vi "testDMA_7858(chunk).vi"() -> ()   [LabVIEW 2020]
uses:
  <vilib>/rvi/Emulation/niFpgaGetClockAttributes.vi
  <vilib>/rvi/Emulation/niFpgaSctlEmulationGetInTimedLoop.vi
  <vilib>/rvi/Emulation/niFpgaEmulationReportErrorSimple.vi
  <vilib>/rvi/DataTransferAndStorage/Container/Common/niFpgaContainerExecOnDevCompGetState.vi
  <vilib>/rvi/errors/niFpgaSetErrorForExecOnDevCompSimple.vi
  <vilib>/rvi/eio/common/nirviEmuReportErrorAndStop.vi
  <vilib>/rvi/interface/RandomDataEmulation/nirviRandomDataAcquireLock.vi
  <vilib>/rvi/interface/RandomDataEmulation/nirviRandomDataQueueStore.vi
  <vilib>/rvi/interface/RandomDataEmulation/nirviRandomDataReleaseLock.vi
  <vilib>/rvi/interface/RandomDataEmulation/nirviFPGAContextMergeError.vi
  <vilib>/rvi/interface/RandomDataEmulation/nirviRandomDataCheckExitLoopConditions.vi
  <vilib>/express/rvi/timingcommon/nirviCommon.vi
  <vilib>/rvi/interface/RandomDataEmulation/niFpgaRandomDataHandleErrors.vi
  <vilib>/rvi/Emulation/niFpgaCriticalErrorInLSC.vi
  <vilib>/rvi/DataTransferAndStorage/Container/XNode/niFpgaContainer.xnode
  <vilib>/rvi/FIFO/Fifo_Resource/niFpgaFifoEmulationRefInMultiElement.vi
panel:
  out "dma read time ticks":u32
  out "write DMA timeout count":i16
  in  "number of samples":i16=100
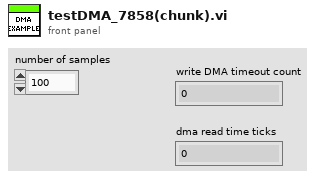
[diagram p1: front panel]
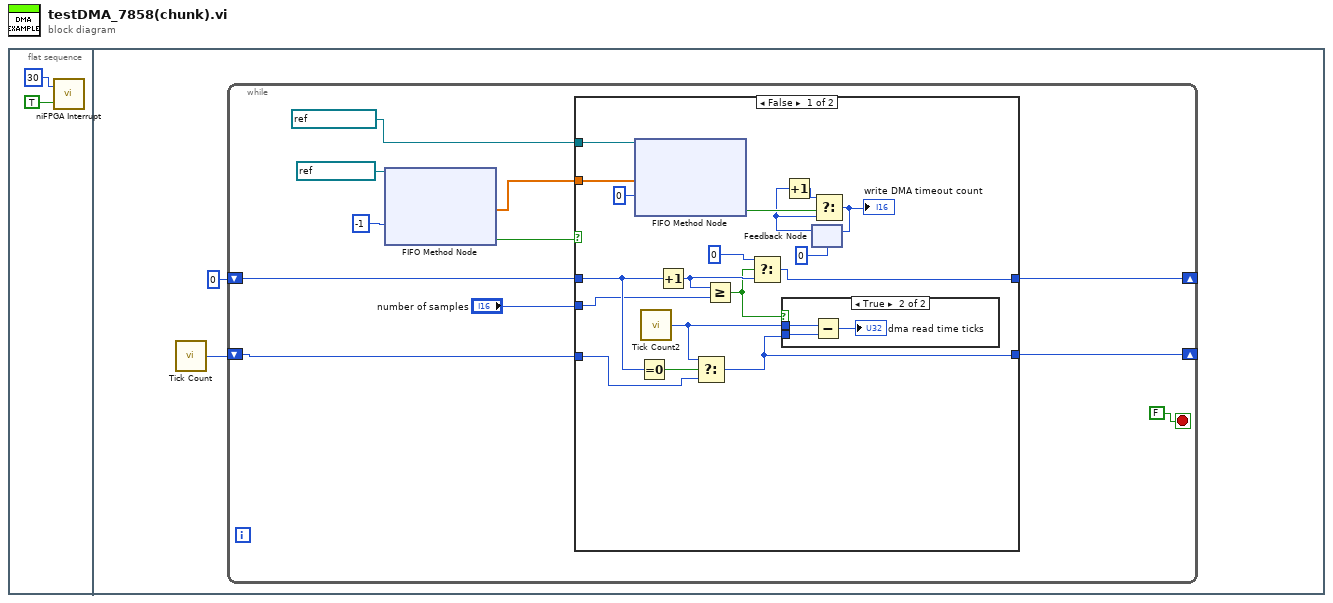
[diagram p0: block diagram]
diagram:
  n1 = flat-sequence {
    frame #0 {
      n2 = call <vilib>:"niFPGA Interrupt.vi"("Wait Until Cleared (F)"=TRUE, "IRQ Number (0)"=u8 30) -> ()  [unwired: 1 in]
    }
    frame #1 {
      n3 = call "Tick Count"() -> ("Tick Count(Ticks)"=w3:u32)
      n4 = while {
        shift-right: [w8] -> _
        shift-left: i16 0 -> [w11]
        shift-right: [w7] -> _
        shift-left: w3 -> [w9]
        stop <- FALSE stop-if-true
        n5 = xnode ("FIFO Method Node")("Timeout"=-1, "FIFO In"=refnum<k21> "Incoming") -> ("Element"=w14:sgl[], "Timed Out?"=w12:bool)  [unwired: 1 out]
        n6 = case shown="False" w12 {
          tunnel: w14 -> [w33 _]
          tunnel: w11 -> [w25 w38]
          tunnel: "number of samples" -> [w24 _]
          tunnel: w9 -> [w20 w37]
          tunnel: [w21 w38] -> w8
          tunnel: [w17 w37] -> w7
          tunnel: refnum<k21> "Outgoing1" ("FIFO In") -> [w16 _]
          frame False {
            n7 = xnode ("FIFO Method Node")("Element"=w33, "Timeout"=0, "FIFO In"=w16) -> ("Timed Out?"=w32:bool)  [unwired: 1 out]
            n8 = Equal To 0?(x=w25) -> (x = 0?=w26:bool)
            n9 = call "Tick Count2"() -> ("Tick Count(Ticks)"=w18:u32)
            n10 = Increment(x=w25) -> (x+1=w22:i16)
            n11 = Select(t=w18, s=w26, f=w20) -> (s? t:f=w17:u32)
            n12 = Greater Or Equal?(x=w22, y=w24) -> (x >= y?=w19:bool)
            n13 = Select(t=i16 0, s=w19, f=w22) -> (s? t:f=w21:i16)
            n14 = case shown="True" w19 {
              tunnel: w18 -> [_ w35]
              tunnel: w17 -> [_ w36]
              frame False {
              }
              frame True {
                n15 = Subtract(x=w35, y=w36) -> (x-y=→"dma read time ticks":u32)
              }
            }
            n16 = feedback #1(i16 0) -> (w30:i16)
            n17 = Increment(x=w30) -> (x+1=w29:i16)
            n18 = Select(t=w29, s=w32, f=w30) -> (s? t:f=w28:i16)
            "write DMA timeout count" <- w28
            n19 = feedback-in #1(w28) -> ()
          }
          frame True {
          }
        }
      }
    }
  }
